vi "WSVCAP SHL FPGA LL I2C Write Data Lines.vi"(0 "Write Bit (U64)":u64, 11 "error in (no error)":errorcluster, 13 "Socket Mask":u64 format="%012x") -> (15 "error out":errorcluster)   [LabVIEW 2012]
uses:
  WSVCAP SHL FPGA LL I2C Debug Global.vi
  <vilib>/eio/EIONode/EIONode.xnode
  <vilib>/rvi/eio/common/nirviEmuTemplateMethod_errors.vi
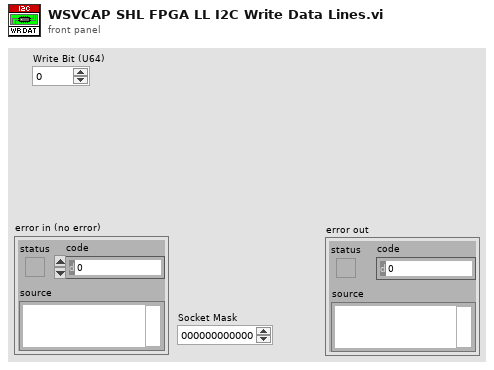
[diagram p1: front panel]
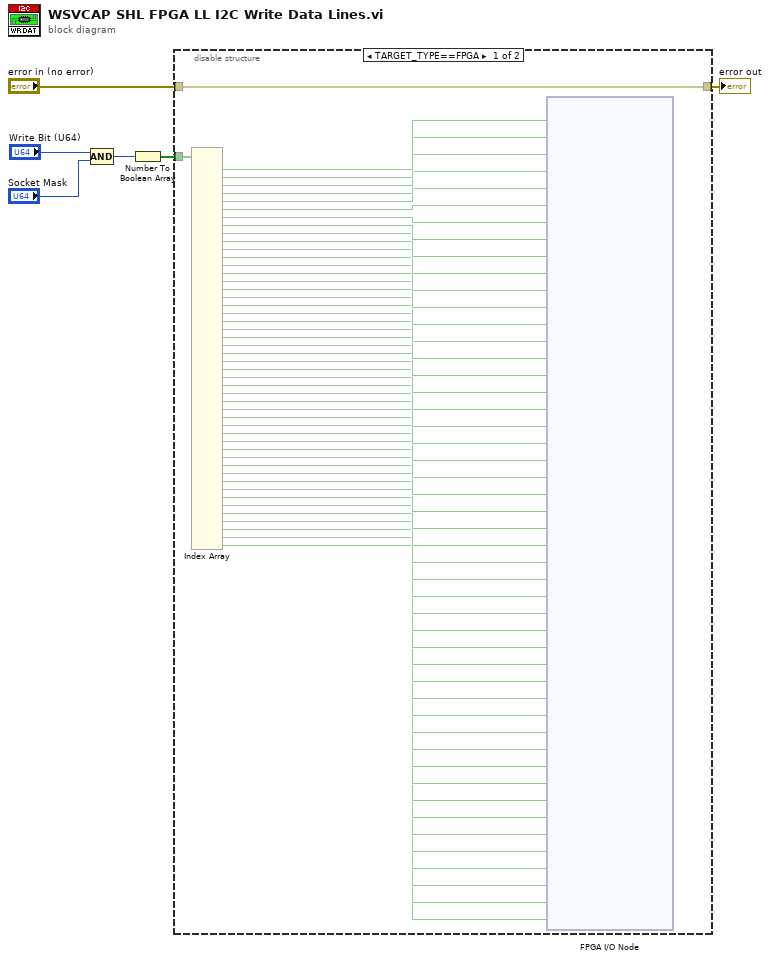
[diagram p0: block diagram]
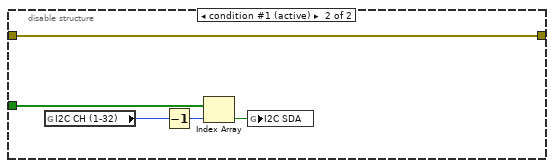
[diagram p2: hidden frame]
diagram:
  n1 = Compound Arithmetic op=AND("Write Bit (U64)", "Socket Mask") -> (w1:u64)
  n2 = Number To Boolean Array(number=w1) -> (Boolean array=w4:bool[])
  n3 = disable-structure shown="TARGET_TYPE==FPGA" {
    disable-tunnel: w4 -> [w7 w60]
    disable-tunnel: [w8 w61] -> w6
    disable-tunnel: "error in (no error)" -> [w8 w61]
    frame condition #0 {
      n4 = Index Array(array=w7) -> (element #1=w56:bool, element #2=w55:bool, element #3=w54:bool, element #4=w53:bool, element #5=w52:bool, element #6=w51:bool, element #7=w50:bool, element #8=w49:bool, element #9=w48:bool, element #10=w47:bool, element #11=w46:bool, element #12=w45:bool, element #13=w44:bool, element #14=w43:bool, element #15=w42:bool, element #16=w41:bool, element #17=w40:bool, element #18=w39:bool, element #19=w38:bool, element #20=w37:bool, element #21=w36:bool, element #22=w35:bool, element #23=w34:bool, element #24=w33:bool, element #25=w32:bool, element #26=w31:bool, element #27=w30:bool, element #28=w29:bool, element #29=w28:bool, element #30=w27:bool, element #31=w26:bool, element #32=w25:bool, element #33=w24:bool, element #34=w23:bool, element #35=w22:bool, element #36=w21:bool, element #37=w20:bool, element #38=w19:bool, element #39=w18:bool, element #40=w17:bool, element #41=w16:bool, element #42=w15:bool, element #43=w14:bool, element #44=w13:bool, element #45=w12:bool, element #46=w11:bool, element #47=w10:bool, element #48=w9:bool)  [unwired: 48 in]
      n5 = xnode "FPGA I/O Node"("I2C_SDA_C1_S1"=w56, "I2C_SDA_C1_S2"=w55, "I2C_SDA_C1_S3"=w54, "I2C_SDA_C1_S4"=w53, "I2C_SDA_C1_S5"=w52, "I2C_SDA_C1_S6"=w51, "I2C_SDA_C1_S7"=w50, "I2C_SDA_C1_S8"=w49, "I2C_SDA_C1_S9"=w48, "I2C_SDA_C1_S10"=w47, "I2C_SDA_C1_S11"=w46, "I2C_SDA_C1_S12"=w45, "I2C_SDA_C1_S13"=w44, "I2C_SDA_C1_S14"=w43, "I2C_SDA_C1_S15"=w42, "I2C_SDA_C1_S16"=w41, "I2C_SDA_C2_S1"=w40, "I2C_SDA_C2_S2"=w39, "I2C_SDA_C2_S3"=w38, "I2C_SDA_C2_S4"=w37, "I2C_SDA_C2_S5"=w36, "I2C_SDA_C2_S6"=w35, "I2C_SDA_C2_S7"=w34, "I2C_SDA_C2_S8"=w33, "I2C_SDA_C2_S9"=w32, "I2C_SDA_C2_S10"=w31, "I2C_SDA_C2_S11"=w30, "I2C_SDA_C2_S12"=w29, "I2C_SDA_C2_S13"=w28, "I2C_SDA_C2_S14"=w27, "I2C_SDA_C2_S15"=w26, "I2C_SDA_C2_S16"=w25, "I2C_SDA_C3_S1"=w24, "I2C_SDA_C3_S2"=w23, "I2C_SDA_C3_S3"=w22, "I2C_SDA_C3_S4"=w21, "I2C_SDA_C3_S5"=w20, "I2C_SDA_C3_S6"=w19, "I2C_SDA_C3_S7"=w18, "I2C_SDA_C3_S8"=w17, "I2C_SDA_C3_S9"=w16, "I2C_SDA_C3_S10"=w15, "I2C_SDA_C3_S11"=w14, "I2C_SDA_C3_S12"=w13, "I2C_SDA_C3_S13"=w12, "I2C_SDA_C3_S14"=w11, "I2C_SDA_C3_S15"=w10, "I2C_SDA_C3_S16"=w9) -> ()  [unwired: 48 in, 48 out]
    }
    frame condition #1 (active) {
      n6 = global read "WSVCAP SHL FPGA LL I2C Debug Global.vi" "I2C CH (1-32)"() -> (w59:i32)
      n7 = Decrement(x=w59) -> (x-1=w57:i32)
      n8 = Index Array(array=w60, index=w57) -> (element=w58:bool)
      n9 = global write "WSVCAP SHL FPGA LL I2C Debug Global.vi" "I2C SDA"(w58) -> ()
    }
  }
  "error out" <- w6
